vi "write string array to file.vi"(8 "error in":errorcluster, 10 "strings":string[](array[string]), 11 "file path":path) -> (0 "error out":errorcluster)   [LabVIEW 2013, in "NISE_CEF_TreeSerializer.lvlib"]
doc: "Writes the full binary contents of a file."
uses:
  NISE_CEF_TreeSerializer.lvlib
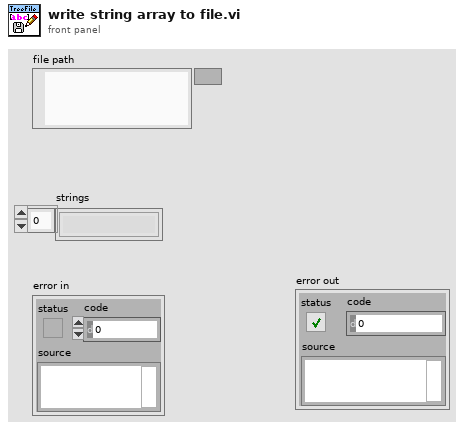
[diagram p1: front panel]
types:
  T1 = enum16{"open", "replace", "create", "open or create", "replace or create", "replace or create with confirmation"}
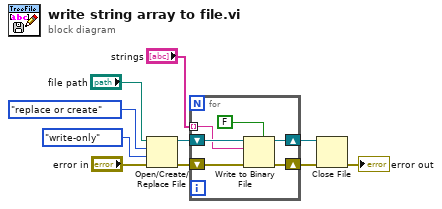
[diagram p0: block diagram]
diagram:
  n1 = Open/Create/Replace File(file path (use dialog)="file path", error in="error in", operation (0:open)=T1."replace or create", access (0:read/write)=enum16{"read/write", "read-only", "write-only"}."write-only") -> (refnum out=w6:refnum<file>, error out=w5:errorcluster)  [unwired: 2 in, 1 out]
  n2 = for {
    shift-right: [w16] -> w10
    shift-left: w6 -> [w14]
    shift-right: [w15] -> w9
    shift-left: w5 -> [w13]
    tunnel: "strings" -> [w11] mode=indexing
    n3 = Write to Binary File(file (use dialog)=w14, data=w11, error in=w13, 5:FALSE ("prepend array or string size? (T)")) -> (refnum out=w16:refnum<file>, error out=w15:errorcluster)  [unwired: 2 in, 1 out]
  }
  n4 = Close File(refnum=w10, error in=w9) -> (error out=→"error out":errorcluster)  [unwired: 1 out]
